vi "Lime.vi"() -> ()   [LabVIEW 2020]
panel:
  out "Shooter Pipeline":dbl
  out "Enabled":bool
  out "Side F/B Drive":dbl
  out "Timer Good":bool
  out "Timer":dbl
  out "Timer Reset":bool
  out "RPM Good":bool
  out "Side F/B Error":dbl
  out "Rotate Error":dbl
  out "F/B Error":dbl
  out "Rotate":dbl
  out "F/B Drive":dbl
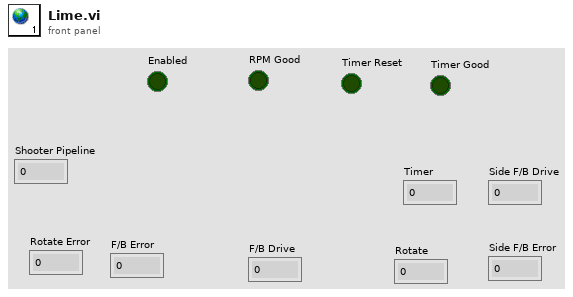
[diagram p1: front panel]
diagram:
